vi "Testing.vi"() -> ()   [LabVIEW 2013]
uses:
  <vilib>/vision/NI_Vision_Development_Module.lvlib
panel:
  out "error out":errorcluster
  out "Particle Features":dbl[][](array[numeric])
  in  "error in":errorcluster
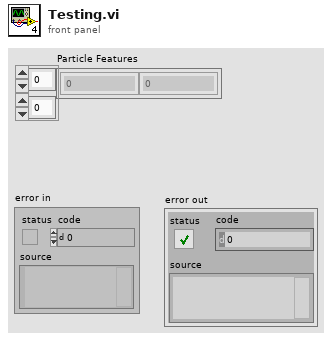
[diagram p1: front panel]
types:
  T1 = typedef "Image Type" = u32
  T2 = typedef "IMAQ Image.ctl" = refnum<image>
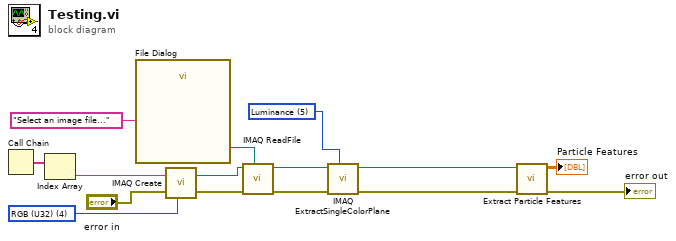
[diagram p0: block diagram]
diagram:
  w7 = 5 items=["Red", "Green", "Blue", "Hue", "Saturation", "Luminance", "Value", "Intensity"] ("Color Plane")
  w8 = T1 4 items=["Grayscale (U8)", "Grayscale (I16)", "Grayscale (SGL)", "Complex (CSG)", "RGB (U32)", "HSL (U32)", "RGB (U64)", "Grayscale (U16)"] ("Image Type")
  n1 = Call Chain() -> (call chain=w12:string[])
  n2 = Index Array(array=w12) -> (element=w11:string)  [unwired: 1 in]
  n3 = call "File Dialog"("prompt"="Select an image file...") -> ("selected path"=w9:path)  [unwired: 6 in, 8 out]
  n4 = call "IMAQ Create"("Image Name"=w11, "Image Type"=w8, "error in (no error)"="error in") -> ("New Image"=w15:T2, "error out"=w14:errorcluster)  [unwired: 1 in, 1 out]
  n5 = call "IMAQ ReadFile"("File Path"=w9, "error in (no error)"=w14, "Image"=w15) -> ("error out"=w5:errorcluster, "Image Out"=w6:T2)  [unwired: 2 in, 5 out]
  n6 = call "IMAQ ExtractSingleColorPlane"("Color Plane"=w7, "error in (no error)"=w5, "Image Src"=w6) -> ("error out"=w4:errorcluster, "Image Dst Out"=w3:T2)  [unwired: 1 in, 6 out]
  n7 = call "Extract Particle Features.vi"("error in (no error)"=w4, "Segment Image"=w3) -> ("error out"=→"error out":errorcluster, "Particle Features"=→"Particle Features":dbl[][])  [unwired: 8 in]
